vi "reset_timeout.vi"(8 "error in (no error)":errorcluster, 11 "Experiment (in)":refnum<class "Experiment.lvclass">) -> (0 "error out":errorcluster, 3 "Experiment":refnum<class "Experiment.lvclass">)   [LabVIEW 2013, in "Experiment.lvclass"]
uses:
  Experiment.lvclass
  Experiment.lvclass/Experiment.ctl
  Globals.vi
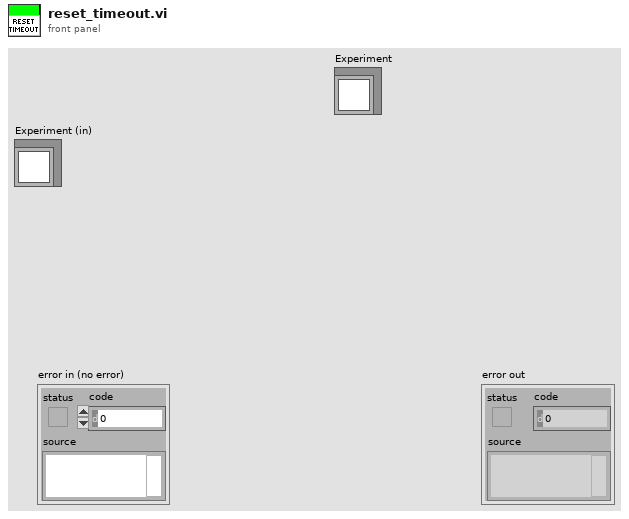
[diagram p1: front panel]
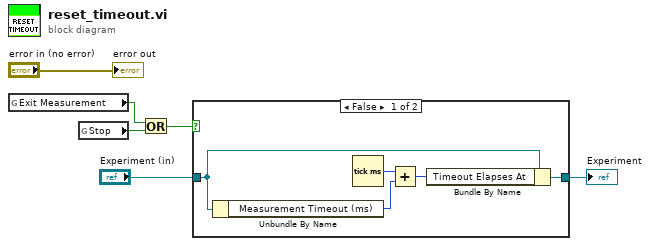
[diagram p0: block diagram]
diagram:
  n1 = global read "Globals.vi" "Exit Measurement"() -> (w5:bool)
  n2 = global read "Globals.vi" "Stop"() -> (w4:bool)
  n3 = Or(x=w5, y=w4) -> (x .or. y?=w3:bool)
  n4 = case shown="False" w3 {
    tunnel: [w11 w12] -> w2
    tunnel: "Experiment (in)" -> [w10 w12]
    frame False {
      n5 = Unbundle By Name(w10) -> ("Measurement Timeout (ms)"=w7:u32)
      n6 = Tick Count (ms)() -> (millisecond timer value=w9:u32)
      n7 = Add(x=w9, y=w7) -> (x+y=w8:u32)
      n8 = Bundle By Name(cluster=w10, "Timeout Elapses At"=w8) -> (w11:refnum<class "Experiment.lvclass">)
    }
    frame True {
    }
  }
  "Experiment" <- w2
  "error out" <- "error in (no error)"
